vi "Test Waveform Flatten.vi"() -> ()   [LabVIEW 2021]
uses:
  typedef/Datatype Waveform.ctl
  CIFfifo.lvclass
  CIFfifo.lvclass/CIFfifo.ctl
  Utilities/Flatten Header.vi
  Flatten/Waveform Flatten.vi/6fdbece9-bad6-4a8e-9bf7-fe1528478dd6.vi
  Flatten/Waveform Flatten.vi/d5e54e4f-7f1a-40ef-960c-6b2cd585230c.vi
  Flatten/Waveform Flatten.vi/a071385d-aa0c-48d2-a5ce-3b08816305e6.vi
  Accessors/Write Payload Length.vi
  Accessors/Read Header.vi
  Utilities/Unflatten Header.vi
  CIFCore/Common/Utilities/Add Error.vi
  Flatten/Waveform Flatten.vi/6fdbece9-bad6-4a8e-9bf7-fe1528478dd6.vi/c28b0ead-42ad-4072-80a2-aca7f2bd7ce3.vi
  Flatten/Waveform Flatten.vi/d5e54e4f-7f1a-40ef-960c-6b2cd585230c.vi/c28b0ead-42ad-4072-80a2-aca7f2bd7ce3.vi
  Flatten/Waveform Flatten.vi/a071385d-aa0c-48d2-a5ce-3b08816305e6.vi/c28b0ead-42ad-4072-80a2-aca7f2bd7ce3.vi
  <vilib>/CIF Foundation/CIF Utilities/Errors/Append Error Location.vi
  ChannelCommon.lvlib
panel:
  in  "Data in":T1[](array[typedef])=[{"measurement"=array[5008 elements], "dT"=0.2, "Timestamp"=215, "Read Lock"=FALSE}, {"measurement"=[0.0, 0.0, 0.0, 0.0, 0.0, 0.0, 0.0, 0.0, 0.0, 0.0, 0.0, 0.0, 0.0, 0.0, 0.0, 0.0, 0.0, 0.0, 0.0, 0.0, 0.0, 0.0, 0.0, 0.0, 0.0, 0.0, 0.0, 0.0, 0.0, 0.0, 0.0, 0.0, 74.0], "dT"=0.366, "Timestamp"=85, "Read Lock"=FALSE}]
  out "Data out":T1[](array[typedef])
  out "error out":errorcluster
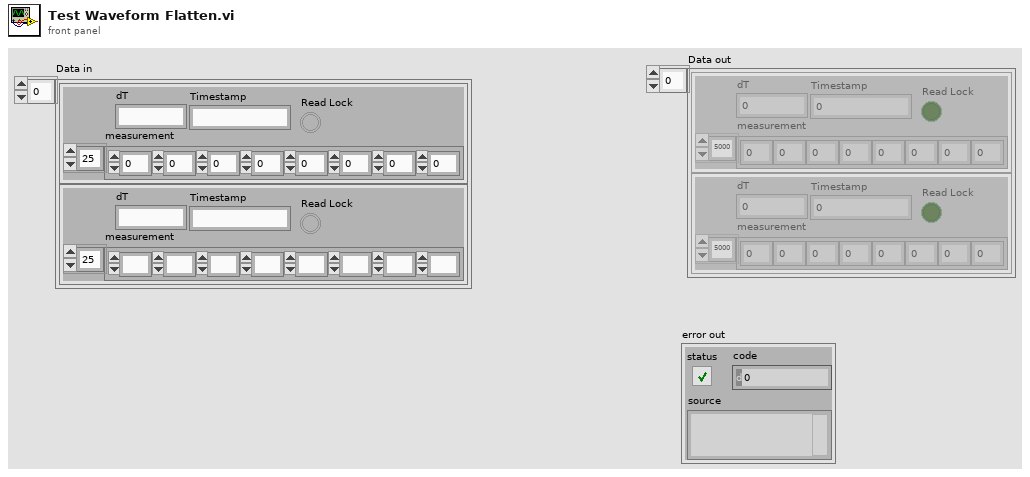
[diagram p1: front panel]
types:
  T1 = typedef "ChannelCommon.lvlib/Datatype Waveform.ctl" = cluster{"measurement":dbl[], "dT":dbl, "Timestamp":u64, "Read Lock":bool}
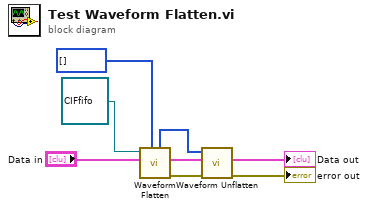
[diagram p0: block diagram]
diagram:
  n1 = call "Waveform Flatten.vi"("payload in"=u8[] [], "Data in"="Data in", "CIFFifo in"=refnum<class "CIFfifo.lvclass"> refnum) -> ("error out"=w8:errorcluster, "Data out"=w1:T1[], "payload out"=w7:u8[])  [unwired: 4 in, 2 out]
  n2 = call "Waveform Unflatten.vi"("error in (no error)"=w8, "Data in in"=w1, "Flatten Data in"=w7) -> ("error out"=→"error out":errorcluster, "Data out"=→"Data out":T1[])  [unwired: 5 in, 2 out]
